vi "Scenario jsObject.vi"(6 "Validate Fields/Templates? (t)":bool=TRUE, 7 "Connection Refnum":T1, 8 "error in (no error)":errorcluster, 9 "Scenario Record (empty)":T2, 10 "Scenario jsObject Name (\"\")":string, 11 "Previous String (\"\")":string) -> (0 "error out":errorcluster, 2 "Scenario jsObject":string, 3 "SCENARIO jsObject Definition":string, 5 "dup Connection Refnum":T1)   [LabVIEW 2011]
uses:
  Scenario Record.ctl
  Conditions/Condition Record.ctl
  Conditions/Condition Operators.ctl
  Summitek EXT/ODBC/SQL Controls/Connection Refnum.ctl
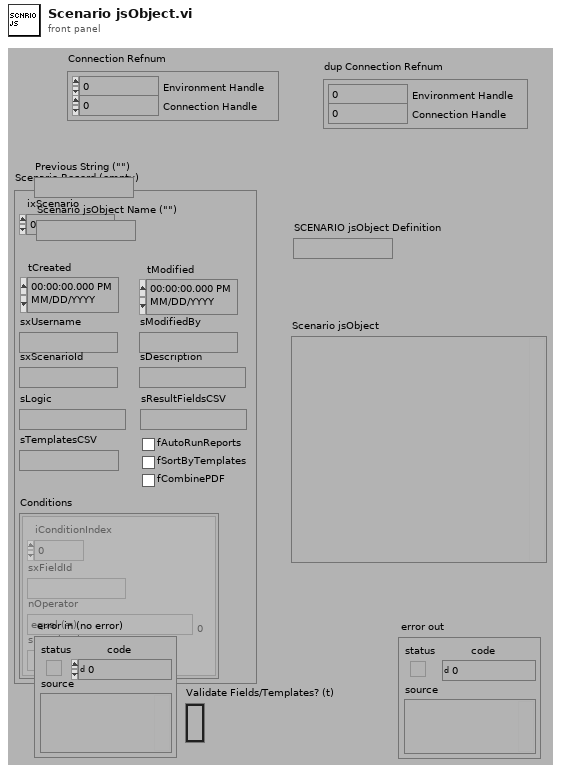
[diagram p1: front panel]
types:
  T1 = typedef "Connection Refnum.ctl" = cluster{"Environment Handle":i32, "Connection Handle":i32}
  T2 = typedef "Scenario Record.ctl" = cluster{"ixScenario":i32, "tCreated":timestamp, "tModified":timestamp, "sxUsername":string, "sModifiedBy":string, "sxScenarioId":string, "sDescription":string, "sLogic":string, "sResultFieldsCSV":string, "sTemplatesCSV":string, "fAutoRunReports":bool, "fSortByTemplates":bool, "fCombinePDF":bool, "Conditions":T3[]}
  T3 = typedef "Condition Record.ctl" = cluster{"iConditionIndex":i32, "sxFieldId":string, "nOperator":T4, "sMatchValue":string}
  T4 = typedef "Condition Operators.ctl" = enum16{"equal (=)", "not equal (\\u2260)", "less than (<)", "less than or equal (\\u2264)", "greater than (>)", "greater than or equal (\\u2265)", "contains", "does not contain"}
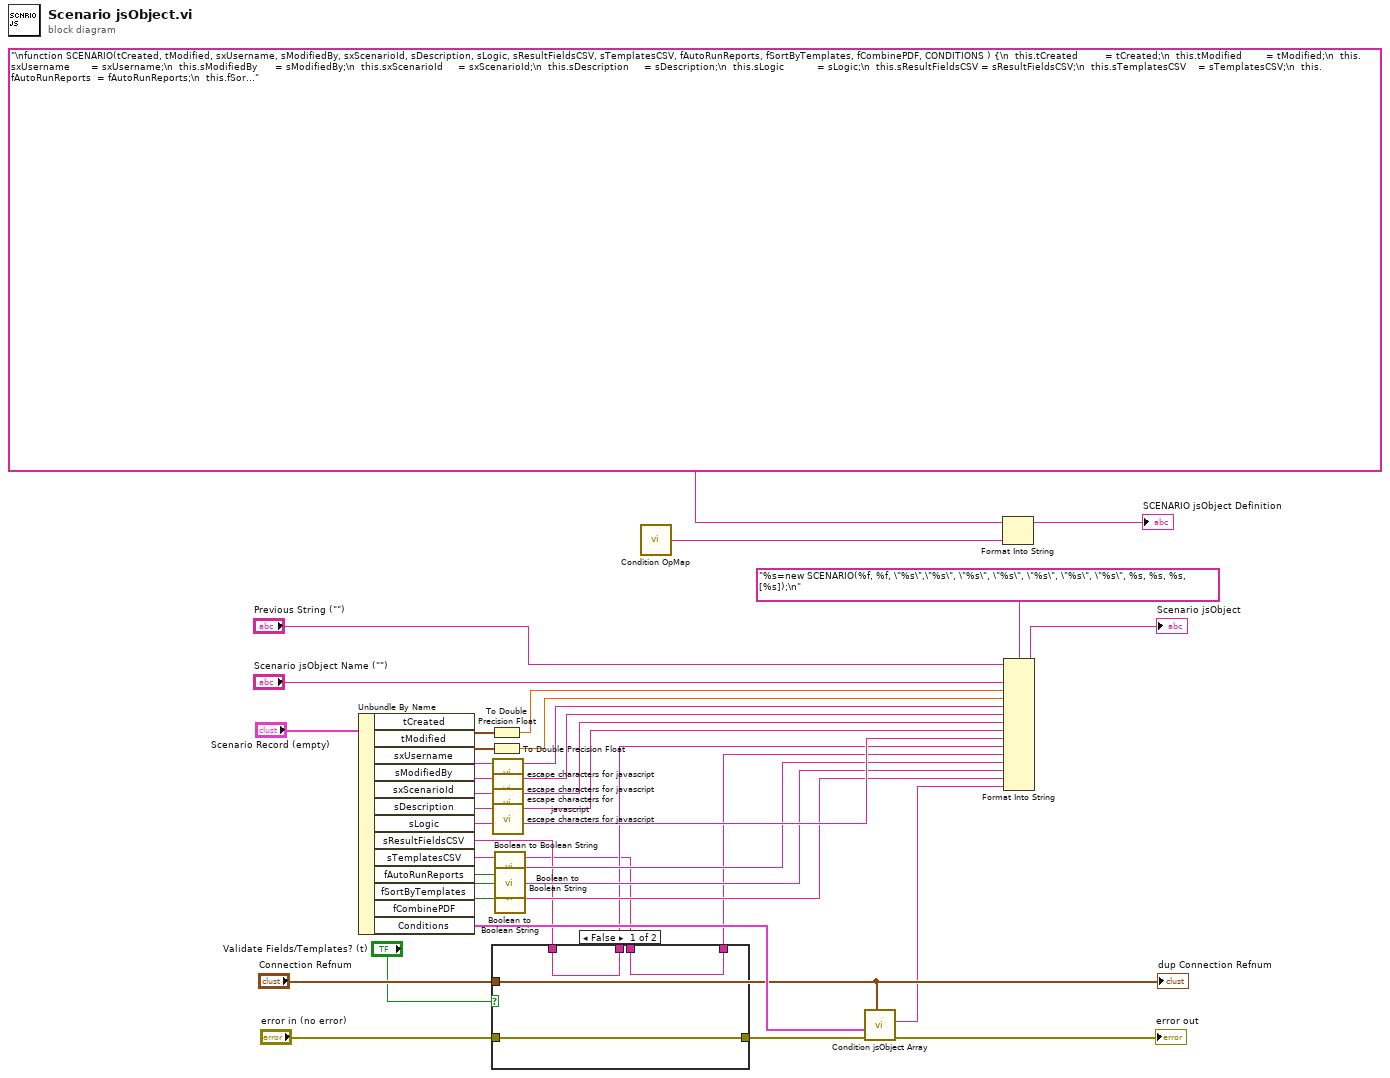
[diagram p0: block diagram]
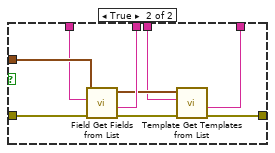
[diagram p2: hidden frame]
diagram:
  n1 = Unbundle By Name("Scenario Record (empty)") -> ("tCreated"=w17:timestamp, "tModified"=w35:timestamp, "sxUsername"=w24:string, "sModifiedBy"=w25:string, "sxScenarioId"=w27:string, "sDescription"=w32:string, "sLogic"=w31:string, "sResultFieldsCSV"=w11:string, "sTemplatesCSV"=w9:string, "fAutoRunReports"=w15:bool, "fSortByTemplates"=w21:bool, "fCombinePDF"=w19:bool, "Conditions"=w29:T3[])
  n2 = To Double Precision Float(number=w17) -> (double precision float=w16:dbl)
  n3 = To Double Precision Float(number=w35) -> (double precision float=w33:dbl)
  n4 = case shown="False" "Validate Fields/Templates? (t)" {
    tunnel: "Connection Refnum" -> [_ w50]
    tunnel: "error in (no error)" -> [w39 w49]
    tunnel: w11 -> [w41 w48]
    tunnel: [w41 w47] -> w10
    tunnel: w9 -> [w40 w45]
    tunnel: [w39 w43] -> w8
    tunnel: [w40 w42] -> w7
    frame False {
    }
    frame True {
      n5 = call "Field Get Fields from List.vi"("error in (no error)"=w49, "sxFieldIdsCSV (\"\")"=w48, "Connection Refnum"=w50) -> ("error out"=w44:errorcluster, "new Fields CSV"=w47:string, "Connection Refnum"=w46:T1)  [unwired: 6 out]
      n6 = call "Template Get Templates from List.vi"("error in (no error)"=w44, "sxTemplateId List(\"\")"=w45, "Connection Refnum"=w46) -> ("error out"=w43:errorcluster, "new Templates CSV"=w42:string)  [unwired: 7 out]
    }
  }
  n7 = call "escape characters for javascript.vi"("String (\"\")"=w24) -> ("escaped String"=w23:string)  [unwired: 4 out]
  n8 = call "escape characters for javascript.vi"("String (\"\")"=w25) -> ("escaped String"=w22:string)  [unwired: 4 out]
  n9 = call "escape characters for javascript.vi"("String (\"\")"=w27) -> ("escaped String"=w26:string)  [unwired: 4 out]
  n10 = call "escape characters for javascript.vi"("String (\"\")"=w32) -> ("escaped String"=w28:string)  [unwired: 4 out]
  n11 = call "Boolean to Boolean String.vi"("Boolean"=w15) -> ("Boolean string"=w14:string)  [unwired: 1 in]
  n12 = call "Boolean to Boolean String.vi"("Boolean"=w21) -> ("Boolean string"=w20:string)  [unwired: 1 in]
  n13 = call "Boolean to Boolean String.vi"("Boolean"=w19) -> ("Boolean string"=w18:string)  [unwired: 1 in]
  n14 = call "Condition OpMap.vi"() -> ("OPERATORS"=w5:string)
  n15 = call "Condition jsObject Array.vi"("Connection Refnum"="Connection Refnum", "error in (no error)"=w8, "CONDITIONS (none)"=w29) -> ("error out"=→"error out":errorcluster, "Conditions jsObject Array"=w4:string)  [unwired: 1 in, 6 out]
  n16 = Format Into String(format string="\nfunction SCENARIO(tCreated, tModified, sxUsername, sModifiedBy, sxScenarioId, sDescription, sLogic, sResultFieldsCSV, sTemplatesCSV, fAutoRunReports, fSortByTemplates, fCombinePDF, CONDITIONS ) {\n  this.tCreated         = tCreated;\n  this.tModified        = tModified;\n  this.sxUsername       = sxUsername;\n  this.sModifiedBy      = sModifiedBy;\n  this.sxScenarioId     = sxScenarioId;\n  this.sDescription     = sDescription;\n  this.sLogic           = sLogic;\n  this.sResultFieldsCSV = sResultFieldsCSV;\n  this.sTemplatesCSV    = sTemplatesCSV;\n  this.fAutoRunReports  = fAutoRunReports;\n  this.fSortByTemplates = fSortByTemplates;\n  this.fCombinePDF      = fCombinePDF;\n\n  this.CONDITIONS       = CONDITIONS;  // array of search condition objects\n  this.OPERATORS        = [%s];        // array of comparison operator objects\n\n  this.TIMESTAMPOPTIONS = [ 'Use date/time', 'Today', 'Yesterday', 'This Week', 'Last Week', 'This Month', 'Last Month', 'This Year', 'Last Year' ];\n\n  this.getOperators     = function(fieldType) {   // array of operators supported by fieldType\n    var s = [];\n    for (var i=0; i<this.OPERATORS.length; i++) {\n      if (this.OPERATORS[i].operatesOn.indexOf(fieldType) >= 0) s.push(this.OPERATORS[i]);\n    }\n    return s;  \n  }\n}\n\n", w5) -> (resulting string=→"SCENARIO jsObject Definition":string)  [unwired: 2 in, 1 out]
  n17 = Format Into String(format string="%s=new SCENARIO(%f, %f, \"%s\",\"%s\", \"%s\", \"%s\", \"%s\", \"%s\", \"%s\", %s, %s, %s, [%s]);\n", initial string="Previous String (\"\")", "Scenario jsObject Name (\"\")", w16, w33, w23, w22, w26, w28, w31, w10, w7, w14, w20, w18, w4) -> (resulting string=→"Scenario jsObject":string)  [unwired: 1 in, 1 out]
  "dup Connection Refnum" <- "Connection Refnum"
